vi "Get Resources (User).vi"(2 "gen":refnum<class "niUSRP Tx DSP v2 FPGA.lvclass">=refnum) -> (3 "fifo.isEmpty":bool, 4 "underflow":bool, 6 "initiate":bool, 8 "abort":bool, 10 "user.gen.fifo":refnum<k21>, 15 "user.clear fifo underflow":refnum<k21>)   [LabVIEW 2023]
doc: "this VI retrieves the start trigger configuration and returns the start trigger value as configured from the host. immediate, software, and digital edge triggers are supported. the trigger is NOT reexported in this VI. \n\n<b>NOTE: software trigger overrides all other behavior.</b>"
uses:
  <vilib>/rvi/DataTransferAndStorage/Container/XNode/niFpgaContainer.xnode
  <vilib>/rvi/DataTransferAndStorage/Register/Emulation/niFpgaRegisterEmulationRefIn.vi
  <instrlib>/niUSRP/Reference FPGA/Tx DSP/niUSRP Tx DSP v2 FPGA.lvclass
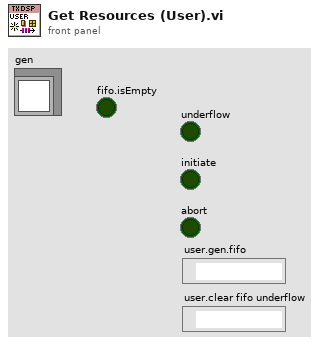
[diagram p1: front panel]
types:
  T1 = typedef "niUSRP Tx DSP v2 FPGA.lvclass/Tx DSP Shared Registers.ctl" = cluster{"reset":refnum<k21>, "reset.done":refnum<k21>, "ignore overflows":refnum<k21>, "overflow":refnum<k21>, "overflow.clear":refnum<k21>, "pipeline delay":refnum<k21>, "group delay (output samples)":refnum<k21>, "blanking delay.data clock ticks":refnum<k21>, "dynamic delay.data clock ticks":refnum<k21>, "dynamic delay.samples":refnum<k21>, "bypass EQ":refnum<k21>, "inject idle into path":refnum<k21>, "TxDspEnabled":refnum<k21>}
  T2 = typedef "niVST Generation Registers v1 FPGA.lvclass/User Registers.ctl" = cluster{"isPlaced":refnum<k21>, "initiate":refnum<k21>, "abort":refnum<k21>, "fifo.clear underflow":refnum<k21>, "fifo.underflow":refnum<k21>, "sampleQuantum":refnum<k21>, "fifo":refnum<k21>, "fifo.empty":refnum<k21>, "fifo.isEmpty":refnum<k21>}
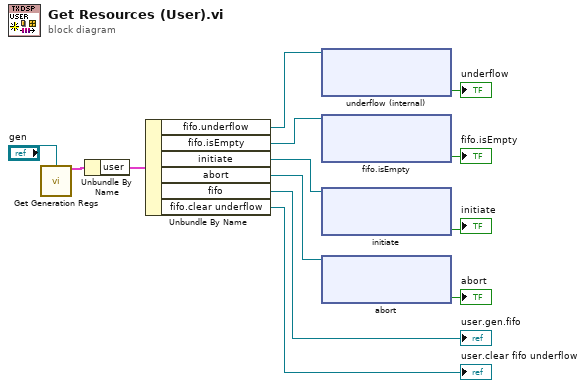
[diagram p0: block diagram]
diagram:
  n1 = call-dynamic "Get Generation Regs.vi"("gen"="gen") -> ("dsp"=w13:T1)  [unwired: 14 in]
  n2 = Unbundle By Name(w13) -> ("user"=w2:T2)
  n3 = Unbundle By Name(w2) -> ("fifo.underflow"=w11:refnum<k21>, "fifo.isEmpty"=w9:refnum<k21>, "initiate"=w10:refnum<k21>, "abort"=w3:refnum<k21>, "fifo"=→"user.gen.fifo":refnum<k21>, "fifo.clear underflow"=→"user.clear fifo underflow":refnum<k21>)
  n4 = xnode "underflow (internal)"("Register In"=w11) -> ("Data"=→"underflow":bool)  [unwired: 1 out]
  n5 = xnode "fifo.isEmpty"("Register In"=w9) -> ("Data"=→"fifo.isEmpty":bool)  [unwired: 1 out]
  n6 = xnode "initiate"("Register In"=w10) -> ("Data"=→"initiate":bool)  [unwired: 1 out]
  n7 = xnode "abort"("Register In"=w3) -> ("Data"=→"abort":bool)  [unwired: 1 out]
